vi "Write Logging Settings.vi"(8 "error in (no error)":errorcluster, 10 "Logging Settings":T1, 11 "Logger Configuration in":refnum<class "Logger Configuration.lvclass">) -> (0 "error out":errorcluster, 3 "Logger Configuration out":refnum<class "Logger Configuration.lvclass">)   [LabVIEW 2017, in "Logger.lvlib" / "Logger Configuration.lvclass"]
uses:
  Logger Configuration.lvclass
  Logger Configuration.lvclass/Logger Configuration.ctl
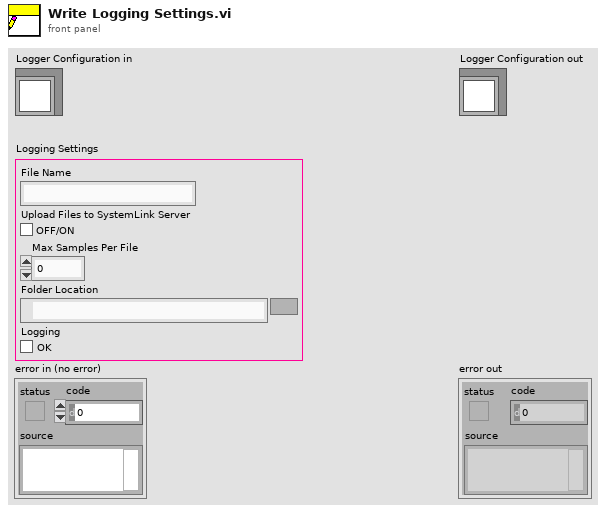
[diagram p1: front panel]
types:
  T1 = cluster{"File Name":string, "Upload Files to SystemLink Server":bool, "Max Samples Per File":i32, "Folder Location":path, "Logging":bool}
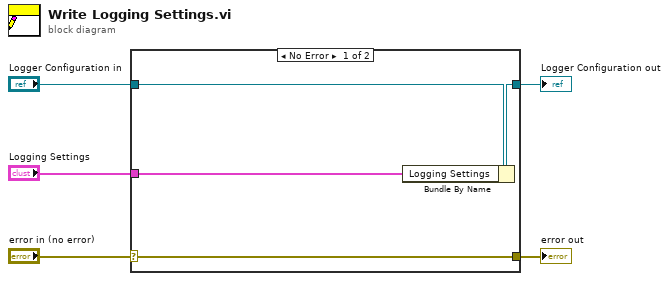
[diagram p0: block diagram]
diagram:
  n1 = case shown="No Error" "error in (no error)" {
    selector: "error in (no error)" -> [w9 w10]
    tunnel: [w9 w10] -> w4
    tunnel: [w7 w11] -> w2
    tunnel: "Logger Configuration in" -> [w8 w11]
    tunnel: "Logging Settings" -> [w6 _]
    frame No Error {
      n2 = Bundle By Name(cluster=w8, "Logging Settings"=w6) -> (w7:refnum<class "Logger Configuration.lvclass">)
    }
    frame Error {
    }
  }
  "error out" <- w4
  "Logger Configuration out" <- w2
